vi "SR830_Messgeraet.vi"(2 "refnum":refnum<file>, 3 "Numerisch":i8 min=0 max=2 step=1) -> ()   [LabVIEW 2019]
uses:
  Global/Global Variables/Data_Display_global.vi
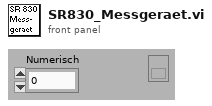
[diagram p1: front panel]
types:
  T1 = typedef "SR830-Cluster.ctl" = cluster{"Lockin 1":dbl[][], "X1-Display":dbl, "Y1-Display":dbl, "X1 Percent":dbl, "X1 Overload":bool, "Y1 Overload":bool, "Unit X1":string, "Unit X2":string, "Unit X2a":string, "Unit X1a":string, "Sensitivity Setpoint":i16, "X1 Percent 2":dbl, "Y1":dbl, "X1":dbl, "Preamp OVL":bool}
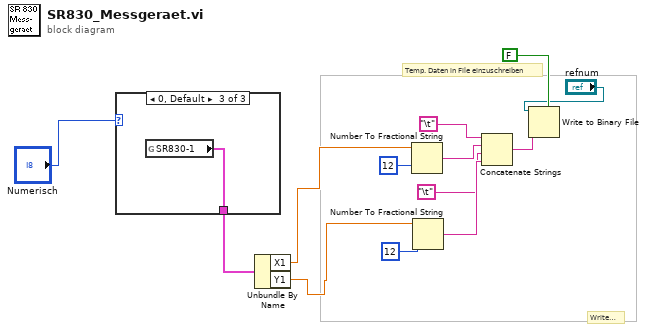
[diagram p0: block diagram]
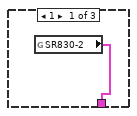
[diagram p2: hidden frame]
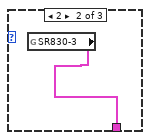
[diagram p3: hidden frame]
diagram:
  # "Temp. Daten in File einzuschreiben"
  # "Write File"
  n1 = case shown="0, Default" "Numerisch" {
    tunnel: [w14 w15 w16] -> w3
    frame 1 {
      n2 = global read "Data_Display_global.vi" "SR830-2"() -> (w14:T1)
    }
    frame 2 {
      n3 = global read "Data_Display_global.vi" "SR830-3"() -> (w15:T1)
    }
    frame 0, Default {
      n4 = global read "Data_Display_global.vi" "SR830-1"() -> (w16:T1)
    }
  }
  n5 = Unbundle By Name(w3) -> ("X1"=w1:dbl, "Y1"=w2:dbl)
  n6 = Number To Fractional String(number=w1, precision (6)=i16 12) -> (F-format string=w11:string)  [unwired: 2 in]
  n7 = Number To Fractional String(number=w2, precision (6)=i16 12) -> (F-format string=w10:string)  [unwired: 2 in]
  n8 = Concatenate Strings("\t", w11, "\t", w10) -> (w13:string)
  n9 = Write to Binary File ("Write File")(file (use dialog)="refnum", data=w13, 5:FALSE ("prepend array or string size? (T)")) -> ()  [unwired: 3 in, 3 out]
